vi "Rename Table.vi"(8 "error in":errorcluster, 9 "New Table Name":string, 10 "Existing Table Name":string, 11 "Data.PG":refnum<class "LV-Data.PGSQL.lvclass">) -> (0 "error out":errorcluster, 2 "SQL":string, 3 "Data.PG out":refnum<class "LV-Data.PGSQL.lvclass">)   [LabVIEW 2016, in "LV-Data.PGSQL.lvclass"]
uses:
  LV-Data.PGSQL.lvclass
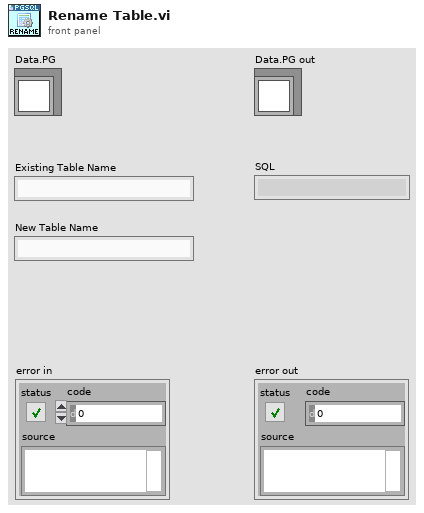
[diagram p1: front panel]
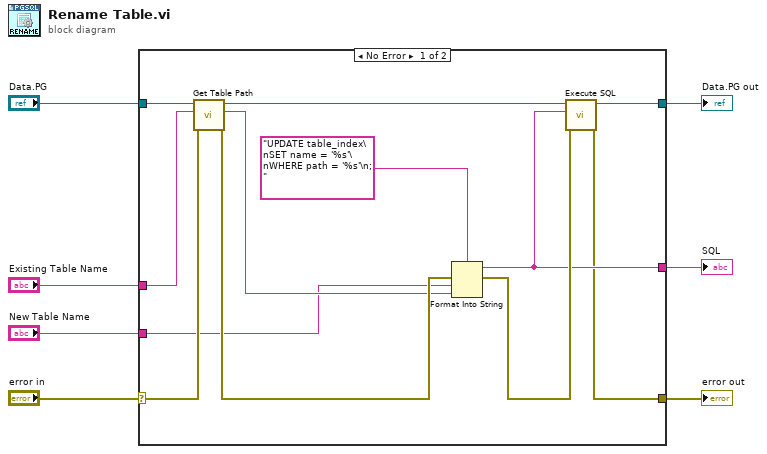
[diagram p0: block diagram]
diagram:
  n1 = case shown="No Error" "error in" {
    selector: "error in" -> [w14 w20]
    tunnel: "Existing Table Name" -> [w15 _]
    tunnel: "New Table Name" -> [w8 _]
    tunnel: [w18 _] -> w5
    tunnel: [w17 w20] -> w4
    tunnel: "Data.PG" -> [w12 w21]
    tunnel: [w16 w21] -> w2
    frame No Error {
      n2 = call "Get Table Path.vi"("error in (no error)"=w14, "Table Name"=w15, "Data.PG"=w12) -> ("error out"=w13:errorcluster, "Table Path"=w9:string, "Data.PG out"=w11:refnum<class "LV-Data.PGSQL.lvclass">)  [unwired: 5 in, 1 out]
      n3 = Format Into String(format string="UPDATE table_index\nSET name = '%s'\nWHERE path = '%s'\n; ", error in=w13, w8, w9) -> (resulting string=w18:string, error out=w19:errorcluster)  [unwired: 1 in]
      n4 = call "Execute SQL.vi"("error in"=w19, "SQL"=w18, "LV-Data.PGSQL"=w11) -> ("error out"=w17:errorcluster, "LV-Data.PGSQL out"=w16:refnum<class "LV-Data.PGSQL.lvclass">)  [unwired: 6 in, 1 out]
    }
    frame Error {
    }
  }
  "SQL" <- w5
  "error out" <- w4
  "Data.PG out" <- w2
